vi "HFRR ADV v13.vi"() -> ()   [LabVIEW 2025] (continued)
              n2120 = String Subset(string=w2617, offset (0)=65, length (rest)=9 ("length (rest)")) -> (substring=w2638:string)
              n2121 = Fract/Exp String To Number(string=w2624) -> (number=w2621:dbl)  [unwired: 3 in, 1 out]
              n2122 = Fract/Exp String To Number(string=w2618) -> (number=w2616:dbl)  [unwired: 3 in, 1 out]
              n2123 = Fract/Exp String To Number(string=w2626) -> (number=w2625:dbl)  [unwired: 3 in, 1 out]
              n2124 = Fract/Exp String To Number(string=w2632) -> (number=w2629:dbl)  [unwired: 3 in, 1 out]
              n2125 = Fract/Exp String To Number(string=w2638) -> (number=w2635:dbl)  [unwired: 3 in, 1 out]
              n2126 = Add(x=w2635, y=0.0) -> (x+y=w2633:dbl)
            }
            n2127 = for {
              N: w2487 -> [_]
              tunnel: w2498 -> [w2578]
              tunnel: w2497 -> [w2577]
              tunnel: [w2567] -> w2456 mode=indexing
              tunnel: [w2565] -> w2454 mode=indexing
              tunnel: [w2566] -> w2450 mode=indexing
              tunnel: w2485 -> [_]
              tunnel: [w2559] -> w2452 mode=indexing
              tunnel: [w2555] -> w2434 mode=indexing
              tunnel: [w2551] -> w2410 mode=indexing
              tunnel: [w2548] -> w2391 mode=indexing
              tunnel: [w2544] -> w2350 mode=indexing
              (unwired) 9 ("length (rest)")
              (unwired) 9 ("length (rest)")
              (unwired) TRUE ("line mode (F)")
              n2128 = Read from Text File "Read File"(file (use dialog)=w2577, error in=w2578) -> (text=w2545:string)  [unwired: 2 in, 3 out]
              n2129 = local write "String 8"(w2545) -> ()
              n2130 = String Subset(string=w2545, offset (0)=85) -> (substring=w2547:string)  [unwired: 1 in]
              n2131 = String Subset(string=w2545, offset (0)=35, length (rest)=9 ("length (rest)")) -> (substring=w2568:string)
              n2132 = String Subset(string=w2545, offset (0)=55, length (rest)=9 ("length (rest)")) -> (substring=w2553:string)
              n2133 = String Subset(string=w2545, offset (0)=25) -> (substring=w2549:string)  [unwired: 1 in]
              n2134 = String Subset(string=w2545, offset (0)=15, length (rest)=9 ("length (rest)")) -> (substring=w2574:string)
              n2135 = String Subset(string=w2545, offset (0)=0, length (rest)=14 ("length (rest)")) -> (substring=w2571:string)
              n2136 = String Subset(string=w2545, offset (0)=45, length (rest)=9 ("length (rest)")) -> (substring=w2558:string)
              n2137 = String Subset(string=w2545, offset (0)=65, length (rest)=9 ("length (rest)")) -> (substring=w2564:string)
              n2138 = Fract/Exp String To Number(string=w2547) -> (number=w2544:dbl)  [unwired: 3 in, 1 out]
              n2139 = Fract/Exp String To Number(string=w2568) -> (number=w2566:dbl)  [unwired: 3 in, 1 out]
              n2140 = Fract/Exp String To Number(string=w2553) -> (number=w2551:dbl)  [unwired: 3 in, 1 out]
              n2141 = Fract/Exp String To Number(string=w2549) -> (number=w2548:dbl)  [unwired: 3 in, 1 out]
              n2142 = Fract/Exp String To Number(string=w2574) -> (number=w2565:dbl)  [unwired: 3 in, 1 out]
              n2143 = Fract/Exp String To Number(string=w2571) -> (number=w2567:dbl)  [unwired: 3 in, 1 out]
              n2144 = Fract/Exp String To Number(string=w2558) -> (number=w2555:dbl)  [unwired: 3 in, 1 out]
              n2145 = Fract/Exp String To Number(string=w2564) -> (number=w2561:dbl)  [unwired: 3 in, 1 out]
              n2146 = Add(x=w2561, y=0.0) -> (x+y=w2559:dbl)
            }
            n2147 = String To Path(string=w2404) -> (path=w2502:path)
            n2148 = String To Path(string=w2402) -> (path=w2496:path)
            n2149 = local read "Numeric 11"() -> (w2486:i32)
            n2150 = local read "Numeric 13"() -> (w2488:i32)
            n2151 = Open/Create/Replace File "Open File"(file path (use dialog)=w2502) -> (refnum out=w2500:refnum<file>, error out=w2499:errorcluster)  [unwired: 5 in, 1 out]
            n2152 = Open/Create/Replace File "Open File"(file path (use dialog)=w2496) -> (refnum out=w2495:refnum<file>, error out=w2494:errorcluster)  [unwired: 5 in, 1 out]
            n2153 = for {
              N: w2486 -> [_]
              tunnel: w2500 -> [w2615]
              tunnel: w2499 -> [w2614]
              tunnel: [w2604] -> w2466 mode=indexing
              tunnel: [w2602] -> w2464 mode=indexing
              tunnel: [w2603] -> w2459 mode=indexing
              tunnel: w2485 -> [_]
              tunnel: [w2596] -> w2461 mode=indexing
              tunnel: [w2592] -> w2437 mode=indexing
              tunnel: [w2588] -> w2412 mode=indexing
              tunnel: [w2584] -> w2393 mode=indexing
              tunnel: [w2579] -> w2351 mode=indexing
              (unwired) TRUE ("line mode (F)")
              n2154 = Read from Text File "Read File"(file (use dialog)=w2615, error in=w2614) -> (text=w2580:string)  [unwired: 2 in, 3 out]
              n2155 = local write "String 7"(w2580) -> ()
              n2156 = String Subset(string=w2580, offset (0)=85, length (rest)=9 ("length (rest)")) -> (substring=w2583:string)
              n2157 = String Subset(string=w2580, offset (0)=35, length (rest)=9 ("length (rest)")) -> (substring=w2605:string)
              n2158 = String Subset(string=w2580, offset (0)=55, length (rest)=9 ("length (rest)")) -> (substring=w2591:string)
              n2159 = String Subset(string=w2580, offset (0)=25, length (rest)=9 ("length (rest)")) -> (substring=w2585:string)
              n2160 = String Subset(string=w2580, offset (0)=45, length (rest)=9 ("length (rest)")) -> (substring=w2593:string)
              n2161 = String Subset(string=w2580, offset (0)=0, length (rest)=14 ("length (rest)")) -> (substring=w2608:string)
              n2162 = String Subset(string=w2580, offset (0)=15, length (rest)=9 ("length (rest)")) -> (substring=w2611:string)
              n2163 = String Subset(string=w2580, offset (0)=65, length (rest)=9 ("length (rest)")) -> (substring=w2597:string)
              n2164 = Fract/Exp String To Number(string=w2583) -> (number=w2579:dbl)  [unwired: 3 in, 1 out]
              n2165 = Fract/Exp String To Number(string=w2605) -> (number=w2603:dbl)  [unwired: 3 in, 1 out]
              n2166 = Fract/Exp String To Number(string=w2591) -> (number=w2588:dbl)  [unwired: 3 in, 1 out]
              n2167 = Fract/Exp String To Number(string=w2585) -> (number=w2584:dbl)  [unwired: 3 in, 1 out]
              n2168 = Fract/Exp String To Number(string=w2593) -> (number=w2592:dbl)  [unwired: 3 in, 1 out]
              n2169 = Fract/Exp String To Number(string=w2608) -> (number=w2604:dbl)  [unwired: 3 in, 1 out]
              n2170 = Fract/Exp String To Number(string=w2611) -> (number=w2602:dbl)  [unwired: 3 in, 1 out]
              n2171 = Fract/Exp String To Number(string=w2597) -> (number=w2600:dbl)  [unwired: 3 in, 1 out]
              n2172 = Add(x=w2600, y=0.0) -> (x+y=w2596:dbl)
            }
            n2173 = for {
              N: w2488 -> [_]
              tunnel: w2495 -> [w2543]
              tunnel: w2494 -> [w2542]
              tunnel: [w2532] -> w2448 mode=indexing
              tunnel: [w2531] -> w2441 mode=indexing
              tunnel: w2485 -> [_]
              tunnel: [w2520] -> w2446 mode=indexing
              tunnel: [w2525] -> w2443 mode=indexing
              tunnel: [w2521] -> w2433 mode=indexing
              tunnel: [w2516] -> w2408 mode=indexing
              tunnel: [w2512] -> w2389 mode=indexing
              tunnel: [w2507] -> w2349 mode=indexing
              (unwired) 1.0 ("x")
              (unwired) TRUE ("line mode (F)")
              n2174 = Read from Text File "Read File"(file (use dialog)=w2543, error in=w2542) -> (text=w2508:string)  [unwired: 2 in, 3 out]
              n2175 = local write "String 12"(w2508) -> ()
              n2176 = String Subset(string=w2508, offset (0)=85, length (rest)=9 ("length (rest)")) -> (substring=w2510:string)
              n2177 = String Subset(string=w2508, offset (0)=35, length (rest)=9 ("length (rest)")) -> (substring=w2533:string)
              n2178 = String Subset(string=w2508, offset (0)=55, length (rest)=9 ("length (rest)")) -> (substring=w2518:string)
              n2179 = String Subset(string=w2508, offset (0)=25, length (rest)=9 ("length (rest)")) -> (substring=w2514:string)
              n2180 = String Subset(string=w2508, offset (0)=45, length (rest)=9 ("length (rest)")) -> (substring=w2523:string)
              n2181 = String Subset(string=w2508, offset (0)=15, length (rest)=9 ("length (rest)")) -> (substring=w2539:string)
              n2182 = String Subset(string=w2508, offset (0)=0, length (rest)=14 ("length (rest)")) -> (substring=w2536:string)
              n2183 = String Subset(string=w2508, offset (0)=65, length (rest)=9 ("length (rest)")) -> (substring=w2526:string)
              n2184 = Fract/Exp String To Number(string=w2510) -> (number=w2507:dbl)  [unwired: 3 in, 1 out]
              n2185 = Fract/Exp String To Number(string=w2533) -> (number=w2531:dbl)  [unwired: 3 in, 1 out]
              n2186 = Fract/Exp String To Number(string=w2518) -> (number=w2516:dbl)  [unwired: 3 in, 1 out]
              n2187 = Fract/Exp String To Number(string=w2514) -> (number=w2512:dbl)  [unwired: 3 in, 1 out]
              n2188 = Fract/Exp String To Number(string=w2523) -> (number=w2521:dbl)  [unwired: 3 in, 1 out]
              n2189 = Fract/Exp String To Number(string=w2539) -> (number=w2520:dbl)  [unwired: 3 in, 1 out]
              n2190 = Fract/Exp String To Number(string=w2536) -> (number=w2532:dbl)  [unwired: 3 in, 1 out]
              n2191 = Fract/Exp String To Number(string=w2526) -> (number=w2529:dbl)  [unwired: 3 in, 1 out]
              n2192 = Add(x=w2529, y=0.0) -> (x+y=w2525:dbl)
            }
            n2193 = Delete From Array(array=w2391, index=0) -> (array with subset deleted=w2364:dbl[])  [unwired: 1 in, 1 out]
            n2194 = Delete From Array(array=w2454, index=0) -> (array with subset deleted=w2427:dbl[])  [unwired: 1 in, 1 out]
            n2195 = Delete From Array(array=w2434, index=0) -> (array with subset deleted=w2422:dbl[])  [unwired: 1 in, 1 out]
            n2196 = Delete From Array(array=w2452, index=0) -> (array with subset deleted=w2453:dbl[])  [unwired: 1 in, 1 out]
            n2197 = call-poly <vilib>:"Mean.vi"("X"=w2364) -> ("mean"=→"КОФ2 4":dbl)  [unwired: 1 out]
            n2198 = call-poly <vilib>:"Mean.vi"("X"=w2427) -> ("mean"=→"КОФ3":dbl)  [unwired: 1 out]
            n2199 = call-poly <vilib>:"Mean.vi"("X"=w2422) -> ("mean"=→"CP3":dbl)  [unwired: 1 out]
            n2200 = Delete From Array(array=w2416, index=0) -> (array with subset deleted=w2343:dbl[])  [unwired: 1 in, 1 out]
            n2201 = Delete From Array(array=w2355, index=0) -> (array with subset deleted=w2342:dbl[])  [unwired: 1 in, 1 out]
            n2202 = Delete From Array(array=w2395, index=0) -> (array with subset deleted=w2366:dbl[])  [unwired: 1 in, 1 out]
            n2203 = Delete From Array(array=w2473, index=0) -> (array with subset deleted=w2428:dbl[])  [unwired: 1 in, 1 out]
            n2204 = Delete From Array(array=w2439, index=0) -> (array with subset deleted=w2424:dbl[])  [unwired: 1 in, 1 out]
            "array w/ subset deleted" <- w2424
            n2205 = Delete From Array(array=w2470, index=0) -> (array with subset deleted=w2471:dbl[])  [unwired: 1 in, 1 out]
            n2206 = call-poly <vilib>:"Mean.vi"("X"=w2366) -> ("mean"=→"КОФ2 2":dbl)  [unwired: 1 out]
            n2207 = call-poly <vilib>:"Mean.vi"("X"=w2428) -> ("mean"=→"КОФ1":dbl)  [unwired: 1 out]
            n2208 = Bundle "Bundle"(w2343, w2342) -> (w2348:cluster{dbl[], dbl[]})  [unwired: 1 in]
            n2209 = Bundle "Bundle"(w2343, w2471) -> (w2335:cluster{dbl[], dbl[]})  [unwired: 1 in]
            n2210 = Delete From Array(array=w2350, index=0) -> (array with subset deleted=w2338:dbl[])  [unwired: 1 in, 1 out]
            n2211 = Delete From Array(array=w2351, index=0) -> (array with subset deleted=w2340:dbl[])  [unwired: 1 in, 1 out]
            n2212 = Delete From Array(array=w2461, index=0) -> (array with subset deleted=w2462:dbl[])  [unwired: 1 in, 1 out]
            n2213 = Delete From Array(array=w2349, index=0) -> (array with subset deleted=w2336:dbl[])  [unwired: 1 in, 1 out]
            n2214 = Delete From Array(array=w2443, index=0) -> (array with subset deleted=w2444:dbl[])  [unwired: 1 in, 1 out]
            n2215 = Delete From Array(array=w2468, index=0) -> (array with subset deleted=w2374:dbl[])  [unwired: 1 in, 1 out]
            n2216 = Delete From Array(array=w2414, index=0) -> (array with subset deleted=w2370:dbl[])  [unwired: 1 in, 1 out]
            n2217 = Delete From Array(array=w2450, index=0) -> (array with subset deleted=w2372:dbl[])  [unwired: 1 in, 1 out]
            n2218 = Delete From Array(array=w2410, index=0) -> (array with subset deleted=w2368:dbl[])  [unwired: 1 in, 1 out]
            n2219 = Delete From Array(array=w2459, index=0) -> (array with subset deleted=w2373:dbl[])  [unwired: 1 in, 1 out]
            n2220 = Delete From Array(array=w2412, index=0) -> (array with subset deleted=w2369:dbl[])  [unwired: 1 in, 1 out]
            n2221 = Delete From Array(array=w2393, index=0) -> (array with subset deleted=w2365:dbl[])  [unwired: 1 in, 1 out]
            n2222 = Delete From Array(array=w2437, index=0) -> (array with subset deleted=w2423:dbl[])  [unwired: 1 in, 1 out]
            n2223 = Delete From Array(array=w2464, index=0) -> (array with subset deleted=w2425:dbl[])  [unwired: 1 in, 1 out]
            n2224 = Delete From Array(array=w2441, index=0) -> (array with subset deleted=w2371:dbl[])  [unwired: 1 in, 1 out]
            n2225 = Delete From Array(array=w2408, index=0) -> (array with subset deleted=w2367:dbl[])  [unwired: 1 in, 1 out]
            n2226 = Delete From Array(array=w2389, index=0) -> (array with subset deleted=w2363:dbl[])  [unwired: 1 in, 1 out]
            n2227 = Delete From Array(array=w2433, index=0) -> (array with subset deleted=w2421:dbl[])  [unwired: 1 in, 1 out]
            n2228 = Delete From Array(array=w2446, index=0) -> (array with subset deleted=w2426:dbl[])  [unwired: 1 in, 1 out]
            n2229 = Delete From Array(array=w2456, index=0) -> (array with subset deleted=w2339:dbl[])  [unwired: 1 in, 1 out]
            n2230 = Delete From Array(array=w2466, index=0) -> (array with subset deleted=w2341:dbl[])  [unwired: 1 in, 1 out]
            n2231 = Delete From Array(array=w2448, index=0) -> (array with subset deleted=w2337:dbl[])  [unwired: 1 in, 1 out]
            n2232 = Bundle "Bundle"(w2343, w2374) -> (w2361:cluster{dbl[], dbl[]})  [unwired: 1 in]
            n2233 = Bundle "Bundle"(w2343, w2428) -> (w2362:cluster{dbl[], dbl[]})  [unwired: 1 in]
            n2234 = Bundle "Bundle"(w2374, w2370) -> (w2376:cluster{dbl[], dbl[]})  [unwired: 1 in]
            n2235 = Bundle "Bundle"(w2339, w2338) -> (w2346:cluster{dbl[], dbl[]})  [unwired: 1 in]
            n2236 = Bundle "Bundle"(w2372, w2368) -> (w2378:cluster{dbl[], dbl[]})  [unwired: 1 in]
            n2237 = Bundle "Bundle"(w2339, w2372) -> (w2482:cluster{dbl[], dbl[]})  [unwired: 1 in]
            n2238 = Bundle "Bundle"(w2339, w2368) -> (w2406:cluster{dbl[], dbl[]})  [unwired: 1 in]
            n2239 = Bundle "Bundle"(w2339, w2427) -> (w2492:cluster{dbl[], dbl[]})  [unwired: 1 in]
            n2240 = Bundle "Bundle"(w2339, w2422) -> (w2430:cluster{dbl[], dbl[]})  [unwired: 1 in]
            n2241 = Bundle "Bundle"(w2339, w2453) -> (w2477:cluster{dbl[], dbl[]})  [unwired: 1 in]
            n2242 = Bundle "Bundle"(w2373, w2369) -> (w2377:cluster{dbl[], dbl[]})  [unwired: 1 in]
            n2243 = Bundle "Bundle"(w2341, w2340) -> (w2347:cluster{dbl[], dbl[]})  [unwired: 1 in]
            n2244 = Bundle "Bundle"(w2341, w2373) -> (w2484:cluster{dbl[], dbl[]})  [unwired: 1 in]
            n2245 = Bundle "Bundle"(w2341, w2369) -> (w2407:cluster{dbl[], dbl[]})  [unwired: 1 in]
            n2246 = Bundle "Bundle"(w2341, w2423) -> (w2431:cluster{dbl[], dbl[]})  [unwired: 1 in]
            n2247 = Bundle "Bundle"(w2341, w2425) -> (w2493:cluster{dbl[], dbl[]})  [unwired: 1 in]
            n2248 = Bundle "Bundle"(w2341, w2462) -> (w2475:cluster{dbl[], dbl[]})  [unwired: 1 in]
            n2249 = Bundle "Bundle"(w2371, w2367) -> (w2379:cluster{dbl[], dbl[]})  [unwired: 1 in]
            n2250 = Bundle "Bundle"(w2337, w2336) -> (w2345:cluster{dbl[], dbl[]})  [unwired: 1 in]
            n2251 = Bundle "Bundle"(w2337, w2371) -> (w2483:cluster{dbl[], dbl[]})  [unwired: 1 in]
            n2252 = Bundle "Bundle"(w2337, w2367) -> (w2405:cluster{dbl[], dbl[]})  [unwired: 1 in]
            n2253 = Bundle "Bundle"(w2337, w2421) -> (w2429:cluster{dbl[], dbl[]})  [unwired: 1 in]
            n2254 = Bundle "Bundle"(w2337, w2426) -> (w2491:cluster{dbl[], dbl[]})  [unwired: 1 in]
            n2255 = Bundle "Bundle"(w2337, w2444) -> (w2476:cluster{dbl[], dbl[]})  [unwired: 1 in]
            n2256 = call-poly <vilib>:"Mean.vi"("X"=w2424) -> ("mean"=→"CP1":dbl)  [unwired: 1 out]
            n2257 = call-poly <vilib>:"Mean.vi"("X"=w2365) -> ("mean"=→"КОФ2 3":dbl)  [unwired: 1 out]
            n2258 = call-poly <vilib>:"Mean.vi"("X"=w2423) -> ("mean"=→"CP2":dbl)  [unwired: 1 out]
            n2259 = call-poly <vilib>:"Mean.vi"("X"=w2425) -> ("mean"=→"КОФ2":dbl)  [unwired: 1 out]
            n2260 = call-poly <vilib>:"Mean.vi"("X"=w2363) -> ("mean"=→"КОФ2 5":dbl)  [unwired: 1 out]
            n2261 = call-poly <vilib>:"Mean.vi"("X"=w2421) -> ("mean"=→"CP4":dbl)  [unwired: 1 out]
            n2262 = call-poly <vilib>:"Mean.vi"("X"=w2426) -> ("mean"=→"КОФ4":dbl)  [unwired: 1 out]
            n2263 = Bundle "Bundle"(w2343, w2370) -> (w2334:cluster{dbl[], dbl[]})  [unwired: 1 in]
            n2264 = Bundle "Bundle"(w2343, w2424) -> (w2357:cluster{dbl[], dbl[]})  [unwired: 1 in]
            n2265 = Build Array "Build Array"(w2334, w2357) -> (w2360:cluster{dbl[], dbl[]}[])
            "XY Graph 17" <- w2360
            n2266 = Build Array "Build Array"(w2348, w2347, w2346, w2345) -> (→"Frequency ( Hz )":cluster{dbl[], dbl[]}[])
            n2267 = Build Array "Build Array"(w2376, w2377, w2378, w2379) -> (→"Air Temp ( °C ) vs Humidity ( % RH )":cluster{dbl[], dbl[]}[])
            n2268 = Build Array "Build Array"(w2361, w2484, w2482, w2483) -> (→"Air Temperature  ( °C )":cluster{dbl[], dbl[]}[])
            n2269 = Build Array "Build Array"(w2334, w2407, w2406, w2405) -> (→"Humidity ( %RH )":cluster{dbl[], dbl[]}[])
            n2270 = Build Array "Build Array"(w2362, w2493, w2492, w2491) -> (→"Coefficient Of Friction":cluster{dbl[], dbl[]}[])
            n2271 = Build Array "Build Array"(w2357, w2431, w2430, w2429) -> (→"Sample Temperature ( °C )":cluster{dbl[], dbl[]}[])
            n2272 = Build Array "Build Array"(w2335, w2475, w2477, w2476) -> (→"XY Graph 13":cluster{dbl[], dbl[]}[])
            n2273 = Bundle "Bundle"(w2343, w2366) -> (w2388:cluster{dbl[], dbl[]})  [unwired: 1 in]
            n2274 = Bundle "Bundle"(w2339, w2364) -> (w2386:cluster{dbl[], dbl[]})  [unwired: 1 in]
            n2275 = Bundle "Bundle"(w2341, w2365) -> (w2387:cluster{dbl[], dbl[]})  [unwired: 1 in]
            n2276 = Bundle "Bundle"(w2337, w2363) -> (w2385:cluster{dbl[], dbl[]})  [unwired: 1 in]
            n2277 = Build Array "Build Array"(w2388, w2387, w2386, w2385) -> (→"Stroke ( mm )":cluster{dbl[], dbl[]}[])
            n2278 = local write "XY Graph 16"(w2360) -> ()
          }
          frame #2 {
          }
          frame #3 {
            n2279 = local write "Numeric 8"(0 ("Numeric 8")) -> ()
            n2280 = local write "Numeric 11"(0 ("Numeric 11")) -> ()
            n2281 = local write "Numeric 12"(0 ("Numeric 12")) -> ()
            n2282 = local write "Numeric 13"(0 ("Numeric 13")) -> ()
            n2283 = property on="OPEN" class="Bool (strict)"("Visible"=TRUE) -> ()  [unwired: 2 in, 2 out]
            n2284 = local read "String Control 2"() -> (w2660:string)
            n2285 = local read "String Control 4"() -> (w2659:string)
            n2286 = local read "String Control 6"() -> (w2658:string)
            n2287 = local read "String Control 8"() -> (w2657:string)
            n2288 = Match Pattern(string=w2660, regular expression="Samples / cycle :- ") -> (after substring=w2674:string)  [unwired: 1 in, 3 out]
            n2289 = Match Pattern(string=w2660, regular expression="Frequency :- ") -> (after substring=w2693:string)  [unwired: 1 in, 3 out]
            n2290 = Match Pattern(string=w2659, regular expression="Samples / cycle :- ") -> (after substring=w2670:string)  [unwired: 1 in, 3 out]
            n2291 = Match Pattern(string=w2659, regular expression="Frequency :- ") -> (after substring=w2688:string)  [unwired: 1 in, 3 out]
            n2292 = Match Pattern(string=w2658, regular expression="Samples / cycle :- ") -> (after substring=w2666:string)  [unwired: 1 in, 3 out]
            n2293 = Match Pattern(string=w2658, regular expression="Frequency :- ") -> (after substring=w2683:string)  [unwired: 1 in, 3 out]
            n2294 = Match Pattern(string=w2657, regular expression="Samples / cycle :- ") -> (after substring=w2662:string)  [unwired: 1 in, 3 out]
            n2295 = Match Pattern(string=w2657, regular expression="Frequency :- ") -> (after substring=w2678:string)  [unwired: 1 in, 3 out]
            n2296 = String Subset(string=w2674, length (rest)=6 ("length (rest)")) -> (substring=w2676:string)  [unwired: 1 in]
            n2297 = String Subset(string=w2693, length (rest)=9 ("length (rest)")) -> (substring=w2695:string)  [unwired: 1 in]
            n2298 = String Subset(string=w2670, length (rest)=6 ("length (rest)")) -> (substring=w2672:string)  [unwired: 1 in]
            n2299 = String Subset(string=w2688, length (rest)=9 ("length (rest)")) -> (substring=w2690:string)  [unwired: 1 in]
            n2300 = String Subset(string=w2666, length (rest)=6 ("length (rest)")) -> (substring=w2668:string)  [unwired: 1 in]
            n2301 = String Subset(string=w2683, length (rest)=9 ("length (rest)")) -> (substring=w2685:string)  [unwired: 1 in]
            n2302 = String Subset(string=w2662, length (rest)=6 ("length (rest)")) -> (substring=w2664:string)  [unwired: 1 in]
            n2303 = String Subset(string=w2678, length (rest)=9 ("length (rest)")) -> (substring=w2680:string)  [unwired: 1 in]
            n2304 = Fract/Exp String To Number(string=w2676) -> (number=w2656:dbl)  [unwired: 3 in, 1 out]
            n2305 = Fract/Exp String To Number(string=w2695) -> (number=w2696:dbl)  [unwired: 3 in, 1 out]
            n2306 = Fract/Exp String To Number(string=w2672) -> (number=w2655:dbl)  [unwired: 3 in, 1 out]
            n2307 = Fract/Exp String To Number(string=w2690) -> (number=w2691:dbl)  [unwired: 3 in, 1 out]
            n2308 = Fract/Exp String To Number(string=w2668) -> (number=w2654:dbl)  [unwired: 3 in, 1 out]
            n2309 = Fract/Exp String To Number(string=w2685) -> (number=w2686:dbl)  [unwired: 3 in, 1 out]
            n2310 = Fract/Exp String To Number(string=w2664) -> (number=w2653:dbl)  [unwired: 3 in, 1 out]
            n2311 = Fract/Exp String To Number(string=w2680) -> (number=w2681:dbl)  [unwired: 3 in, 1 out]
            n2312 = local write "sample1"(w2656) -> ()
            n2313 = local write "freq1"(w2696) -> ()
            n2314 = local write "sample2"(w2655) -> ()
            n2315 = local write "freq2"(w2691) -> ()
            n2316 = local write "sample3"(w2654) -> ()
            n2317 = local write "freq3"(w2686) -> ()
            n2318 = local write "sample4"(w2653) -> ()
            n2319 = local write "freq 4"(w2681) -> ()
          }
        }
      }
    }
    n2320 = case shown="True" w2143 {
      selector: w2143 -> [_ w2272]
      frame False {
      }
      frame True {
        n2321 = Not(x=w2272) -> (.not. x?=w2268:bool)
        n2322 = local write "service 3"(w2268) -> ()
        n2323 = local write "OPEN 6"(w2268) -> ()
        n2324 = call <vilib>:"System Exec.vi"("wait until completion? (T)"=TRUE, "command line"="C:\\LAB-IQ\\Scar View.exe") -> ("error out"=→"error out 5":errorcluster)  [unwired: 6 in, 3 out]
      }
    }
    n2325 = case shown="\"Acquire\", Default" w2155 {
      frame "Acquire", Default {
        w3195 = 0.2 ("y")
        w3200 = 1.0 ("y")
        w3201 = 0.8 ("y")
        # "Elapsed time\ncof\nstroke\nAir temp\nTemp\nHumidity"
        n2326 = disable-structure shown="Disabled" {
          frame Disabled {
            n2327 = local read "Flag"() -> (w3218:dbl)
            n2328 = local read "RUN"() -> (w3215:bool)
            n2329 = Not(x=w3215) -> (.not. x?=w3214:bool)
            n2330 = Equal?(x=w3218, y=10.0) -> (x = y?=w3216:bool)
            n2331 = And(x=w3216, y=w3214) -> (x .and. y?=w3213:bool)
            n2332 = case shown="True" w3213 {
              frame False {
              }
              frame True {
                w3219 = FALSE ("Heater Button")
                n2333 = local write "Humidity"(w3219) -> ()
                n2334 = local write "Heater Button"(w3219) -> ()
              }
            }
          }
          frame Enabled {
          }
        }
        n2335 = disable-structure shown="Disabled" {
          frame Disabled {
            n2336 = case shown="True" {
              selector: _ -> [_ _]
              frame False {
              }
              frame True {
                w3310 = TRUE ("Heater")
                n2337 = local write "Humidity"(w3310) -> ()
                n2338 = local write "Heater Button"(w3310) -> ()
                n2339 = local read "TEST STANDARD"() -> (w3313:T3)
                n2340 = local read "TEST STANDARD"() -> (w3308:T3)
                n2341 = Equal?(x=w3313, y=enum16{"ASTM D6079", "ISO 12156", "Custom"}."ISO 12156" ("Test Standard")) -> (x = y?=w3311:bool)
                n2342 = Equal?(x=w3308, y=enum16{"ASTM D6079", "ISO 12156", "Custom"}."ASTM D6079" ("Test Standard")) -> (x = y?=w3307:bool)
                n2343 = case shown="True" w3311 {
                  frame False {
                  }
                  frame True {
                    n2344 = local write "Heater"(TRUE ("Heater")) -> ()
                    n2345 = local write "airtempflg"(FALSE ("airtempflg")) -> ()
                  }
                }
                n2346 = case shown="True" w3307 {
                  frame False {
                  }
                  frame True {
                    n2347 = local write "Heater"(FALSE ("Heater")) -> ()
                    n2348 = local write "airtempflg"(TRUE ("airtempflg")) -> ()
                  }
                }
              }
            }
          }
          frame Enabled {
          }
        }
        n2349 = stacked-sequence {
          frame #0 {
            n2350 = case shown="True" "RST FF" {
              frame False {
              }
              frame True {
                w3376 = 0.0 ("X Scale.Range:Maximum")
                n2351 = property on="Frictional Force ( N )" class="WFChart (strict)"("XScale.Maximum"=600.0 ("X Scale.Range:Maximum"), "XScale.Minimum"=w3376, "YScale.Maximum"=10.0 ("Y Scale.Range:Maximum"), "YScale.Minimum"=w3376) -> ()  [unwired: 2 in, 2 out]
              }
            }
          }
          frame #1 {
            n2352 = case shown="True" "RST TEMP" {
              frame False {
              }
              frame True {
                n2353 = property on="Temperature ( Deg C )" class="WFChart (strict)"("XScale.Minimum"=0.0 ("X Scale.Range:Minimum"), "XScale.Maximum"=600.0 ("X Scale.Range:Maximum"), "YScale.Minimum"=0.0 ("Y Scale.Range:Minimum"), "YScale.Maximum"=100.0 ("Y Scale.Range:Maximum")) -> ()  [unwired: 2 in, 2 out]
              }
            }
          }
          frame #2 {
            n2354 = case shown="True" "RSTCOF" {
              frame False {
              }
              frame True {
                n2355 = property on="Coefficient of Friction" class="WFChart (strict)"("XScale.Minimum"=0.0 ("X Scale.Range:Minimum"), "XScale.Maximum"=600.0 ("X Scale.Range:Maximum"), "YScale.Maximum"=1.0 ("X Scale.Range:Minimum"), "YScale.Minimum"=0.0 ("X Scale.Range:Minimum")) -> ()  [unwired: 2 in, 2 out]
              }
            }
          }
          frame #3 {
            n2356 = case shown="True" "RSTCOF 2" {
              frame False {
              }
              frame True {
                (unwired) 100.0 ("Y Scale.Range:Maximum")
                (unwired) 0.0 ("Y Scale.Range:Minimum")
                (unwired) 600.0 ("X Scale.Range:Maximum")
                (unwired) 0.0 ("X Scale.Range:Minimum")
              }
            }
          }
          frame #4 {
            n2357 = case shown="True" "RSTCOF 3" {
              frame False {
              }
              frame True {
                n2358 = property on="Electrical Contact Resistance ( % )" class="WFChart (strict)"("XScale.Minimum"=0.0 ("X Scale.Range:Minimum"), "XScale.Maximum"=600.0 ("X Scale.Range:Maximum"), "YScale.Minimum"=0.0 ("Y Scale.Range:Minimum"), "YScale.Maximum"=100.0 ("Y Scale.Range:Maximum")) -> ()  [unwired: 2 in, 2 out]
              }
            }
          }
        }
        n2359 = disable-structure shown="Disabled" {
          frame Disabled {
            n2360 = case shown="True" {
              selector: _ -> [_ _]
              frame False {
              }
              frame True {
                n2361 = local read "zflag 2"() -> (w3277:dbl)
                n2362 = local read "yflag"() -> (w3279:dbl)
                n2363 = Equal?(x=w3279, y=2.0 ("tflag")) -> (x = y?=w3281:bool)
                n2364 = Equal?(x=w3277, y=3.0 ("tflag")) -> (x = y?=w3280:bool)
                n2365 = And(x=w3281, y=w3280) -> (x .and. y?=w3275:bool)
                n2366 = case shown="True" w3275 {
                  frame False {
                  }
                  frame True {
                    w3306 = 0.0 ("zflag")
                    n2367 = local write "zflag"(w3306) -> ()
                    n2368 = local write "zflag 2"(w3306) -> ()
                    n2369 = Delete(path (use dialog)=path "C:/LAB-IQ-NXT/WO 2449 TT.sig" ("file path (dialog if empty)")) -> (deleted path=w3305:path)  [unwired: 4 in, 2 out]
                    n2370 = Delete(path (use dialog)=path "C:/LAB-IQ-NXT/WO 2449 TRH.sig" ("file path (dialog if empty)")) -> (deleted path=w3300:path)  [unwired: 4 in, 2 out]
                    n2371 = local read "SEN.RUN HRS"() -> (w3292:dbl)
                    n2372 = local read "SENSOR TIME"() -> (w3290:dbl)
                    n2373 = call <vilib>:"compatOverwrite.vi"("overwrite (F)"=TRUE) -> ("overwrite?"=w3282:T26)
                    n2374 = call <vilib>:"compatOverwrite.vi"("overwrite (F)"=TRUE) -> ("overwrite?"=w3286:T26)
                    n2375 = local read "Total No. of Tests"() -> (w3293:dbl)
                    n2376 = Add(x=w3290, y=w3292) -> (x+y=w3291:dbl)
                    "SEN.RUN HRS" <- w3291
                    n2377 = Open/Create/Replace File(file path (use dialog)=w3305, operation (0:open)=w3282) -> (refnum out=w3283:refnum<file>, error out=w3284:errorcluster)  [unwired: 4 in, 1 out]
                    n2378 = Open/Create/Replace File(file path (use dialog)=w3300, operation (0:open)=w3286) -> (refnum out=w3287:refnum<file>, error out=w3288:errorcluster)  [unwired: 4 in, 1 out]
                    n2379 = Deny Access(4:w3284, 6:T24."deny none" ("deny mode (2)"), 7:w3283) -> (3:w3304:refnum<file>)  [unwired: 1 out]
                    n2380 = Deny Access(4:w3288, 6:T24."deny none" ("deny mode (2)"), 7:w3287) -> (3:w3296:refnum<file>)  [unwired: 1 out]
                    n2381 = Number To Decimal String(number=w3293) -> (decimal integer string=w3301:string)  [unwired: 1 in]
                    n2382 = Number To Decimal String(number=w3291) -> (decimal integer string=w3297:string)  [unwired: 1 in]
                    n2383 = Write to Binary File(file (use dialog)=w3304, data=w3301, 5:FALSE ("prepend array or string size? (T)")) -> ()  [unwired: 3 in, 3 out]
                    n2384 = Write to Binary File(file (use dialog)=w3296, data=w3297, 5:FALSE ("prepend array or string size? (T)")) -> ()  [unwired: 3 in, 3 out]
                  }
                }
              }
            }
          }
          frame Enabled {
          }
        }
        n2385 = local read "RUN"() -> (w3204:bool)
        n2386 = local read "run replace"() -> (w3208:bool)
        n2387 = local read "run replace"() -> (w3207:bool)
        n2388 = case shown="True" w3204 {
          frame False {
            n2389 = local write "run replace"(FALSE ("run replace")) -> ()
          }
          frame True {
            "run replace" <- TRUE ("run replace")
          }
        }
        n2390 = local read "RUN"() -> (w3212:bool)
        n2391 = local read "Set Temp"() -> (w3174:dbl)
        n2392 = local read "SetTemp"() -> (w3176:dbl)
        n2393 = case shown="False" w3212 {
          tunnel: [FALSE ("TEST RUNNING") TRUE ("TEST RUNNING")] -> w3211
          frame False {
            w3395 = 0.0 ("Flag")
            n2394 = local write "Elapsed time"(0.0 ("elapsedtime")) -> ()
            n2395 = local write "Time Remaining"(w3395) -> ()
            n2396 = local write "Flag"(w3395) -> ()
            n2397 = local write "Remaining Time"(w3395) -> ()
          }
          frame True {
            n2398 = local write "Flag"(10.0 ("Flag")) -> ()
          }
        }
        n2399 = case shown="False" w3208 {
          frame False {
            n2400 = local read "zflag"() -> (→"zflag 2":dbl)
            n2401 = local write "yflag"(2.0 ("tflag")) -> ()
            n2402 = local write "FLAG 4"(0.0 ("FLAG")) -> ()
          }
          frame True {
            n2403 = local write "yflag"(1.0 ("tflag")) -> ()
            n2404 = local write "zflag"(3.0 ("zflag")) -> ()
          }
        }
        n2405 = local read "acq 2"() -> (w3206:bool)
        n2406 = local read "AIR TEMP"() -> (w3169:dbl)
        n2407 = local read "Amb temp"() -> (w3173:dbl)
        n2408 = case shown="True" "Save & Continue" {
          frame False {
          }
          frame True {
            "acq 2" <- TRUE ("acq 2")
          }
        }
        n2409 = local read "Set Rh"() -> (w3175:dbl)
        n2410 = Add(x=w3176, y=w3201) -> (x+y=w3202:dbl)
        n2411 = Subtract(x=w3176, y=w3201) -> (x-y=w3203:dbl)
        n2412 = Add(x=w3174, y=w3195) -> (x+y=w3196:dbl)
        n2413 = Subtract(x=w3174, y=w3195) -> (x-y=w3197:dbl)
        n2414 = And(x=w3206, y=w3207) -> (x .and. y?=w3205:bool)
        n2415 = Greater Or Equal?(x=w3169, y=15.0) -> (x >= y?=w3170:bool)
        "powstat" <- w3170
        n2416 = local read "Humidity ( %RH )"() -> (w3172:dbl)
        n2417 = case shown="True" "Save & Continue" {
          frame False {
          }
          frame True {
            n2418 = while {
              tunnel: "0123456789abcdefghijklmnopqrstuvwxyzABCDEFGHIJKLMNOPQRSTUVWXYZ" ("string 2") -> [w3366]
              shift-right: [w3364] -> w3359
              shift-left: "" -> [w3363]
              i -> [w3373]
              stop <- w3372 stop-if-true
              n2419 = Random Number (0-1)() -> (number: 0 to 1=w3367:dbl)
              n2420 = Multiply(x=w3367, y=62.0) -> (x*y=w3369:dbl)
              n2421 = Decrement(x="Length") -> (x-1=w3362:i16)
              n2422 = To Word Integer(number=w3369) -> (16bit integer=w3370:i16)
              n2423 = String Subset(string=w3366, offset (0)=w3370, length (rest)=1 ("length (rest)")) -> (substring=w3365:string)
              n2424 = Greater Or Equal?(x=w3373, y=w3362) -> (x >= y?=w3372:bool)
              n2425 = Concatenate Strings(w3365, w3363) -> (w3364:string)
            }
            n2426 = local write "UUID"(w3359) -> ()
          }
        }
        n2427 = In Range and Coerce(upper limit=w3202, x=w3173, lower limit=w3203) -> (In Range?=w3192:bool)  [unwired: 1 out]
        n2428 = Add(x=w3175, y=w3200) -> (x+y=w3199:dbl)
        n2429 = Subtract(x=w3175, y=w3200) -> (x-y=w3198:dbl)
        n2430 = local read "TEMP"() -> (w3171:dbl)
        n2431 = case shown="True" "Save & Continue" {
          frame False {
          }
          frame True {
            n2432 = local read "Operator ID"() -> (w3715:string)
            n2433 = local read "FILE"() -> (w3721:string)
            n2434 = String Length(string=w3721) -> (length=w3719:i32)
            n2435 = String Length(string=w3715) -> (length=w3716:i32)
            n2436 = Greater?(x=w3719, y=0) -> (0:w3718:bool)
            n2437 = Greater?(x=w3716, y=0) -> (0:w3714:bool)
            n2438 = And(x=w3718, y=w3714) -> (x .and. y?=w3713:bool)
            n2439 = case shown="True" w3713 {
              frame False {
                n2440 = stacked-sequence {
                  frame #0 {
                    n2441 = One Button Dialog(message="Please Enter a File Name and Operator ID to save data !", button name ("OK")="Ok") -> ()  [unwired: 1 out]
                  }
                  frame #1 {
                    n2442 = local write "Save & Continue"(FALSE ("OK Button")) -> ()
                  }
                }
                n2443 = local write "Save & Continue"(FALSE ("OK Button")) -> ()
              }
              frame True {
                n2444 = stacked-sequence {
                  frame #0 {
                    n2445 = local read "FILE"() -> (w3727:string)
                    n2446 = call "file check.vi"("file name in"=w3727) -> ("file name out"=w3726:string)  [unwired: 9 in, 1 out]
                    n2447 = call <vilib>:"Application Directory.vi"() -> ("Application Directory"=w3737:path)
                    n2448 = Build Path(base path=w3737, name or relative path="data") -> (appended path=w3736:path)
                    n2449 = call <vilib>:"Trim Whitespace.vi"("string"=w3726) -> ("trimmed string"=w3734:string)  [unwired: 1 in]
                    n2450 = call <vilib>:"Trim Whitespace.vi"("string"=w3726) -> ("trimmed string"=w3735:string)  [unwired: 1 in]
                    n2451 = List Folder(path=w3736) -> (folder names=w3732:string[])  [unwired: 3 in, 3 out]
                    n2452 = Match Pattern(string=w3734, regular expression="_(") -> (before substring=w3731:string)  [unwired: 1 in, 3 out]
                    n2453 = for {
                      tunnel: w3732 -> [w3746] mode=indexing
                      tunnel: w3731 -> [w3744]
                      shift-right: [w3742] -> w3729
                      shift-left: bool[] [] -> [w3743]
                      n2454 = Match Pattern(string=w3746, regular expression="_(") -> (before substring=w3745:string)  [unwired: 1 in, 3 out]
                      n2455 = Equal?(x=w3745, y=w3744) -> (x = y?=w3741:bool)
                      n2456 = case shown="True" w3741 {
                        tunnel: w3741 -> [_ w3749]
                        tunnel: w3743 -> [w3748 w3751]
                        tunnel: [w3748 w3750] -> w3742
                        frame False {
                        }
                        frame True {
                          n2457 = Insert Into Array(array=w3751, new element=w3749) -> (w3750:bool[])  [unwired: 1 in]
                        }
                      }
                    }
                    n2458 = Equal?(x=w3732, y=w3731) -> (x = y?=w3740:bool[])
                    n2459 = Or Array Elements(Boolean array=w3740) -> (logical OR=w3739:bool)
                    n2460 = Array Size(array=w3729) -> (size(s)=w3728:i32)
                    n2461 = case shown="True" w3739 {
                      tunnel: w3735 -> [_ w3759]
                      tunnel: w3728 -> [_ w3752]
                      frame False {
                      }
                      frame True {
                        n2462 = Number To Decimal String(number=w3752) -> (decimal integer string=w3755:string)  [unwired: 1 in]
                        n2463 = Search/Split String(string=w3759, search string/char (-)="_(" ("regular expression")) -> (substring before match=w3757:string)  [unwired: 1 in, 2 out]
                        n2464 = Concatenate Strings(w3757, "_(" ("regular expression"), w3755, ")" ("regular expression")) -> (w3753:string)
                        n2465 = local write "FILE"(w3753) -> ()
                      }
                    }
                  }
                  frame #1 {
                    w3761 = 0.0
                    w3774 = cluster{"y":dbl, dbl, "y":dbl}[] [] ("History Data")
                    w3775 = FALSE ("Heater Button")
                    (unwired) ")!" ("string")
                    (unwired) ")" ("string")
                    w3773 = dbl[] [] ("History Data")
                    w3779 = "\r"
                    # "C:\\WinDucom\\Data\\"
                    # "C:\\LAB-IQ-NXT\\data"
                    n2466 = local write "Humidity ( %RH )"(w3761) -> ()
                    n2467 = local write "Frequency ( Hz )"(w3761) -> ()
                    n2468 = local write "Stroke 3"(w3761) -> ()
                    n2469 = local write "speedop"(0.0 ("PIDclk 2")) -> ()
                    n2470 = local write "Set Temp 2"(65.0 ("Set Temp 2")) -> ()
                    n2471 = local write "AIR TEMP"(w3761) -> ()
                    n2472 = local write "clk"(0.0 ("clk")) -> ()
                    n2473 = local write "Stroke 4"(w3761) -> ()
                    n2474 = local write "Stroke"(w3761) -> ()
                    n2475 = local write "COF 3"(w3761) -> ()
                    n2476 = local write "COF 2"(w3761) -> ()
                    n2477 = local write "TEMP"(w3761) -> ()
                    n2478 = local write "ecr 3"(w3761) -> ()
                    n2479 = local write "FF 3"(w3761) -> ()
                    n2480 = local write "FF 2"(w3761) -> ()
                    n2481 = property on="Humidity ( %RH )" class="WFChart (strict)"("History Data"=w3773) -> ()  [unwired: 2 in, 2 out]
                    n2482 = property on="Coefficient of Friction" class="WFChart (strict)"("History Data"=w3773) -> ()  [unwired: 2 in, 2 out]
                    n2483 = property on="Coefficient of Friction" class="WFChart (strict)"("History Data"=w3773) -> ()  [unwired: 2 in, 2 out]
                    n2484 = property on="Frictional Force ( N )" class="WFChart (strict)"("History Data"=w3773) -> ()  [unwired: 2 in, 2 out]
                    n2485 = property on="Electrical Contact Resistance ( % )" class="WFChart (strict)"("History Data"=w3773) -> ()  [unwired: 2 in, 2 out]
                    n2486 = property on="Electrical Contact Resistance ( % )" class="WFChart (strict)"("History Data"=w3773) -> ()  [unwired: 2 in, 2 out]
                    n2487 = property on="Temperature ( Deg C )" class="WFChart (strict)"("History Data"=w3773) -> ()  [unwired: 2 in, 2 out]
                    n2488 = property on="Frictional Force ( N )" class="WFChart (strict)"("History Data"=w3773) -> ()  [unwired: 2 in, 2 out]
                    n2489 = property on="Coefficient of Friction" class="WFChart (strict)"("History Data"=w3773) -> ()  [unwired: 2 in, 2 out]
                    n2490 = property on="Frictional Force ( N )" class="WFChart (strict)"("History Data"=w3773) -> ()  [unwired: 2 in, 2 out]
                    n2491 = property on="Electrical Contact Resistance ( % )" class="WFChart (strict)"("History Data"=w3773) -> ()  [unwired: 2 in, 2 out]
                    n2492 = property on="Temperature ( Deg C )" class="WFChart (strict)"("History Data"=w3773) -> ()  [unwired: 2 in, 2 out]
                    n2493 = property on="Humidity ( %RH )" class="WFChart (strict)"("History Data"=w3773) -> ()  [unwired: 2 in, 2 out]
                    n2494 = property on="Stroke ( mm )" class="WFChart (strict)"("History Data"=w3774) -> ()  [unwired: 2 in, 2 out]
                    n2495 = property on="Stroke ( mm )" class="WFChart (strict)"("History Data"=w3774) -> ()  [unwired: 2 in, 2 out]
                    n2496 = local write "Humidity"(w3775) -> ()
                    n2497 = local write "Heater Button"(w3775) -> ()
                    n2498 = local read "FILE"() -> (w3769:string)
                    n2499 = disable-structure shown="Enabled" {
                      disable-tunnel: [w3814 _] -> w3760
                      frame Enabled {
                        n2500 = local read "NORMAL LOAD"() -> (w3814:dbl)
                      }
                      frame Disabled {
                      }
                    }
                    n2501 = call "file check.vi"("file name in"=w3769) -> ("error out"=w3772:errorcluster, "file name out"=w3766:string)  [unwired: 9 in]
                    n2502 = call "FILE PATH CREATION.vi"("error in"=w3772, "FILE NAME :"=w3766) -> ("FILE OUT"=w3765:path)  [unwired: 8 in, 1 out]
                    n2503 = Concatenate Strings(w3766, ".dgf" ("Substring")) -> (w3771:string)
                    n2504 = Concatenate Strings(w3766, ".duf" ("Substring")) -> (w3767:string)
                    n2505 = Multiply(x=w3760, y=1.0) -> (x*y=w3793:dbl)
                    n2506 = Build Path(base path=w3765, name or relative path=w3771) -> (appended path=w3764:path)
                    n2507 = Build Path(base path=w3765, name or relative path=w3767) -> (appended path=w3763:path)
                    n2508 = Number To Fractional String(number=w3793, width (-)=i16 5, precision (6)=i16 2) -> (F-format string=w3801:string)  [unwired: 1 in]
                    n2509 = local read "Fuel Discription :"() -> (w3789:string)
                    n2510 = local read "Batch Ref Num :"() -> (w3777:string)
                    n2511 = Get Date/Time String(date format (0)=enum16{"short", "long", "abbreviated"}."short") -> (date string=w3812:string, time string=w3809:string)  [unwired: 2 in]
                    n2512 = local read "Remarks :"() -> (w3788:string)
                    n2513 = Concatenate Strings("Load :- " ("Substring"), w3801, " grams ," ("Substring")) -> (w3800:string)
                    n2514 = local read "String 41"() -> (w3780:string)
                    n2515 = Concatenate Strings(w3789) -> (w3790:string)
                    n2516 = Concatenate Strings(w3777) -> (w3776:string)
                    n2517 = Concatenate Strings("tested by") -> (w3784:string)
                    n2518 = Concatenate Strings("(" ("Substring"), w3812, ")" ("Substring"), w3809) -> (w3782:string)
                    "concatenated string" <- w3782
                    n2519 = Concatenate Strings(w3788, "," ("string")) -> (w3787:string)
                    n2520 = Concatenate Strings("  TIME;      COF;       STROKE;     AIR TEMP;  TEMP;  HUMIDITY;  ECR; PID-OUT; FREQUENCY" ("Substring"), "\r") -> (w3796:string)
                    n2521 = Concatenate Strings(w3780, w3779, "Fuel Discription :-" ("Substring"), w3790, w3779, w3800, w3779, "Batch Ref Num :-" ("Substring"), w3776, w3779, " Remarks :- " ("Substring"), w3787, w3779, " Date :- " ("Substring"), w3782, w3779, "Tested By :-" ("Substring"), w3784) -> (w3794:string)
                    "REMARKS" <- w3794
                    n2522 = call <vilib>:"Write Characters To File.vi"("append to file? (new file:F)"=FALSE, "character string"=w3796, "file path (dialog if empty)"=w3764) -> ()  [unwired: 2 in, 1 out]
                    n2523 = call <vilib>:"Write Characters To File.vi"("append to file? (new file:F)"=FALSE, "character string"=w3794, "file path (dialog if empty)"=w3763) -> ()  [unwired: 2 in, 1 out]
                  }
                  frame #2 {
                    n2524 = local write "Cycles elapsed"(0 ("Cycles elapsed")) -> ()
                    n2525 = local write "cyclecount"(0 ("cyclecount")) -> ()
                    n2526 = local write "Save & Continue"(FALSE ("OK")) -> ()
                    n2527 = local write "autostrtflg"(TRUE ("autostrtflg")) -> ()
                    n2528 = local write "Save"(FALSE ("Save")) -> ()
                    n2529 = Get Date/Time In Seconds() -> (seconds since 1Jan1904=w3819:timestamp)
                    n2530 = To Double Precision Float(number=w3819) -> (double precision float=w3818:dbl)
                    n2531 = local write "acq timer"(w3818) -> ()
                    n2532 = One Button Dialog(message="Please ensure sample is mounted properly and machine is ready in all aspects for testing !", button name ("OK")="Ok") -> ()  [unwired: 1 out]
                  }
                  frame #3 {
                    n2533 = stacked-sequence {
                      frame #0 {
                        n2534 = local write "Main Dashboard Buttons"(T1."Dashboard" ("Main Dashboard Buttons")) -> ()
                        n2535 = local write "Main Tab"(T2."Acquire" ("Main Tab")) -> ()
                      }
                      frame #1 {
                        n2536 = local write "EVENT LOG"("" ("EVENT LOG")) -> ()
                      }
                      frame #2 {
                        n2537 = Wait (ms)(milliseconds to wait=u32 50) -> ()  [unwired: 1 out]
                      }
                      frame #3 {
                        n2538 = disable-structure shown="Disabled" {
                          frame Disabled {
                            n2539 = local read "EVENT LOG"() -> (w3831:string)
                            n2540 = call "Event Log.vi"("Content"="Test Details", "EVENT LOG"=w3831) -> ("EVENT LOG"=w3830:string)  [unwired: 8 in, 1 out]
                            n2541 = local write "EVENT LOG"(w3830) -> ()
                          }
                          frame Enabled {
                          }
                        }
                      }
                      frame #4 {
                        n2542 = Wait (ms)(milliseconds to wait=u32 50) -> ()  [unwired: 1 out]
                      }
                      frame #5 {
                        n2543 = local read "FILE"() -> (w3833:string)
                        n2544 = Concatenate Strings("File Name :" ("Content"), w3833) -> (w3834:string)
                        n2545 = local read "EVENT LOG"() -> (w3837:string)
                        n2546 = call "Event Log.vi"("Content"=w3834, "EVENT LOG"=w3837) -> ("EVENT LOG"=w3836:string)  [unwired: 8 in, 1 out]
                        n2547 = local write "EVENT LOG"(w3836) -> ()
                      }
                      frame #6 {
                        n2548 = Wait (ms)(milliseconds to wait=u32 50) -> ()  [unwired: 1 out]
                      }
                      frame #7 {
                        n2549 = local read "Batch Ref Num :"() -> (w3839:string)
                        n2550 = Concatenate Strings("Batch Ref No :" ("Content"), w3839) -> (w3840:string)
                        n2551 = local read "EVENT LOG"() -> (w3843:string)
                        n2552 = call "Event Log.vi"("Content"=w3840, "EVENT LOG"=w3843) -> ("EVENT LOG"=w3842:string)  [unwired: 8 in, 1 out]
                        n2553 = local write "EVENT LOG"(w3842) -> ()
                      }
                      frame #8 {
                        n2554 = Wait (ms)(milliseconds to wait=u32 50) -> ()  [unwired: 1 out]
                      }
                      frame #9 {
                        n2555 = local read "tested by"() -> (w3845:string)
                        n2556 = Concatenate Strings("Tested By :" ("Content"), w3845) -> (w3846:string)
                        n2557 = local read "EVENT LOG"() -> (w3849:string)
                        n2558 = call "Event Log.vi"("Content"=w3846, "EVENT LOG"=w3849) -> ("EVENT LOG"=w3848:string)  [unwired: 8 in, 1 out]
                        n2559 = local write "EVENT LOG"(w3848) -> ()
                      }
                      frame #10 {
                        n2560 = Wait (ms)(milliseconds to wait=u32 50) -> ()  [unwired: 1 out]
                      }
                      frame #11 {
                        n2561 = local read "TEST STANDARD"() -> (w3852:T3)
                        n2562 = case shown="\"ASTM D6079\", Default" w3852 {
                          tunnel: ["ASTM D6079" "ISO 12156" "CEC F-096-A-06" "Custom"] -> w3851
                          frame "ASTM D6079", Default {
                          }
                          frame "ISO 12156" {
                          }
                          frame "CEC F-096-A-06" {
                          }
                          frame "Custom" {
                          }
                        }
                        n2563 = Concatenate Strings("Test Standard :" ("Content"), w3851) -> (w3853:string)
                        n2564 = local read "EVENT LOG"() -> (w3856:string)
                        n2565 = call "Event Log.vi"("Content"=w3853, "EVENT LOG"=w3856) -> ("EVENT LOG"=w3855:string)  [unwired: 8 in, 1 out]
                        n2566 = local write "EVENT LOG"(w3855) -> ()
                      }
                      frame #12 {
                        n2567 = Wait (ms)(milliseconds to wait=u32 50) -> ()  [unwired: 1 out]
                      }
                      frame #13 {
                        n2568 = local read "Fuel Discription :"() -> (w3862:string)
                        n2569 = Concatenate Strings("Fuel Description :" ("Content"), w3862) -> (w3863:string)
                        n2570 = local read "EVENT LOG"() -> (w3866:string)
                        n2571 = call "Event Log.vi"("Content"=w3863, "EVENT LOG"=w3866) -> ("EVENT LOG"=w3865:string)  [unwired: 8 in, 1 out]
                        n2572 = local write "EVENT LOG"(w3865) -> ()
                      }
                      frame #14 {
                        n2573 = Wait (ms)(milliseconds to wait=u32 50) -> ()  [unwired: 1 out]
                      }
                      frame #15 {
                        n2574 = local read "Remarks :"() -> (w3868:string)
                        n2575 = Concatenate Strings("Remarks :" ("Content"), w3868) -> (w3869:string)
                        n2576 = local read "EVENT LOG"() -> (w3872:string)
                        n2577 = call "Event Log.vi"("Content"=w3869, "EVENT LOG"=w3872) -> ("EVENT LOG"=w3871:string)  [unwired: 8 in, 1 out]
                        n2578 = local write "EVENT LOG"(w3871) -> ()
                      }
                      frame #16 {
                        n2579 = Wait (ms)(milliseconds to wait=u32 50) -> ()  [unwired: 1 out]
                      }
                      frame #17 {
                        n2580 = local read "Operator ID"() -> (w3874:string)
                        n2581 = Concatenate Strings("Operator ID :" ("Content"), w3874) -> (w3876:string)
                        n2582 = local read "EVENT LOG"() -> (w3878:string)
                        n2583 = call "Event Log.vi"("Content"=w3876, "EVENT LOG"=w3878) -> ("EVENT LOG"=w3877:string)  [unwired: 8 in, 1 out]
                        n2584 = local write "EVENT LOG"(w3877) -> ()
                      }
                      frame #18 {
                        n2585 = Wait (ms)(milliseconds to wait=u32 50) -> ()  [unwired: 1 out]
                      }
                      frame #19 {
                        n2586 = disable-structure shown="Disabled" {
                          frame Disabled {
                            n2587 = local read "EVENT LOG"() -> (w3882:string)
                            n2588 = call "Event Log.vi"("Content"="Test Parameter", "EVENT LOG"=w3882) -> ("EVENT LOG"=w3881:string)  [unwired: 8 in, 1 out]
                            n2589 = local write "EVENT LOG"(w3881) -> ()
                          }
                          frame Enabled {
                          }
                        }
                      }
                      frame #20 {
                        n2590 = Wait (ms)(milliseconds to wait=u32 50) -> ()  [unwired: 1 out]
                      }
                      frame #21 {
                        n2591 = local read "Set Hz"() -> (w3886:dbl)
                        n2592 = Number To Fractional String(number=w3886, precision (6)=i16 2) -> (F-format string=w3885:string)  [unwired: 2 in]
                        n2593 = Concatenate Strings("Set Frequency [Hz] :" ("Content"), w3885) -> (w3888:string)
                        n2594 = local read "EVENT LOG"() -> (w3890:string)
                        n2595 = call "Event Log.vi"("Content"=w3888, "EVENT LOG"=w3890) -> ("EVENT LOG"=w3889:string)  [unwired: 8 in, 1 out]
                        n2596 = local write "EVENT LOG"(w3889) -> ()
                      }
                      frame #22 {
                        n2597 = Wait (ms)(milliseconds to wait=u32 50) -> ()  [unwired: 1 out]
                      }
                      frame #23 {
                        n2598 = local read "NORMAL LOAD"() -> (w3893:dbl)
                        n2599 = Number To Fractional String(number=w3893, precision (6)=i16 2) -> (F-format string=w3894:string)  [unwired: 2 in]
                        n2600 = Concatenate Strings("Applied Load [grams] :" ("Content"), w3894) -> (w3896:string)
                        n2601 = local read "EVENT LOG"() -> (w3898:string)
                        n2602 = call "Event Log.vi"("Content"=w3896, "EVENT LOG"=w3898) -> ("EVENT LOG"=w3897:string)  [unwired: 8 in, 1 out]
                        n2603 = local write "EVENT LOG"(w3897) -> ()
                      }
                      frame #24 {
                        n2604 = Wait (ms)(milliseconds to wait=u32 50) -> ()  [unwired: 1 out]
                      }
                      frame #25 {
                        n2605 = local read "Set Strk"() -> (w3901:dbl)
                        n2606 = Number To Fractional String(number=w3901, precision (6)=i16 2) -> (F-format string=w3902:string)  [unwired: 2 in]
                        n2607 = Concatenate Strings("Set Stroke [mm] :" ("Content"), w3902) -> (w3904:string)
                        n2608 = local read "EVENT LOG"() -> (w3906:string)
                        n2609 = call "Event Log.vi"("Content"=w3904, "EVENT LOG"=w3906) -> ("EVENT LOG"=w3905:string)  [unwired: 8 in, 1 out]
                        n2610 = local write "EVENT LOG"(w3905) -> ()
                      }
                      frame #26 {
                        n2611 = Wait (ms)(milliseconds to wait=u32 50) -> ()  [unwired: 1 out]
                      }
                      frame #27 {
                        n2612 = local read "Set Temp"() -> (w3909:dbl)
                        n2613 = Number To Fractional String(number=w3909, precision (6)=i16 2) -> (F-format string=w3910:string)  [unwired: 2 in]
                        n2614 = Concatenate Strings("Set Temperature [deg C] :" ("Content"), w3910) -> (w3912:string)
                        n2615 = local read "EVENT LOG"() -> (w3914:string)
                        n2616 = call "Event Log.vi"("Content"=w3912, "EVENT LOG"=w3914) -> ("EVENT LOG"=w3913:string)  [unwired: 8 in, 1 out]
                        n2617 = local write "EVENT LOG"(w3913) -> ()
                      }
                      frame #28 {
                        n2618 = Wait (ms)(milliseconds to wait=u32 50) -> ()  [unwired: 1 out]
                      }
                      frame #29 {
                        n2619 = local read "Set Rh"() -> (w3917:dbl)
                        n2620 = Number To Fractional String(number=w3917, precision (6)=i16 2) -> (F-format string=w3918:string)  [unwired: 2 in]
                        n2621 = Concatenate Strings("Set Humidity [%RH] :" ("Content"), w3918) -> (w3920:string)
                        n2622 = local read "EVENT LOG"() -> (w3922:string)
                        n2623 = call "Event Log.vi"("Content"=w3920, "EVENT LOG"=w3922) -> ("EVENT LOG"=w3921:string)  [unwired: 8 in, 1 out]
                        n2624 = local write "EVENT LOG"(w3921) -> ()
                      }
                      frame #30 {
                        n2625 = Wait (ms)(milliseconds to wait=u32 50) -> ()  [unwired: 1 out]
                      }
                      frame #31 {
                        n2626 = local read "test time"() -> (w3925:dbl)
                        n2627 = Number To Fractional String(number=w3925, precision (6)=i16 1) -> (F-format string=w3926:string)  [unwired: 2 in]
                        n2628 = Concatenate Strings("Test Duration [mins] :" ("Content"), w3926) -> (w3928:string)
                        n2629 = local read "EVENT LOG"() -> (w3930:string)
                        n2630 = call "Event Log.vi"("Content"=w3928, "EVENT LOG"=w3930) -> ("EVENT LOG"=w3929:string)  [unwired: 8 in, 1 out]
                        n2631 = local write "EVENT LOG"(w3929) -> ()
                      }
                      frame #32 {
                        w3931 = dbl[] [] ("History Data")
                        w3932 = cluster{"y":dbl, dbl, "y":dbl}[] [] ("History Data")
                        w3933 = FALSE ("Visible")
                        n2632 = property on="Stroke ( mm )" class="WFChart (strict)"("History Data"=w3932) -> ()  [unwired: 2 in, 2 out]
                        n2633 = property on="Humidity ( %RH )" class="WFChart (strict)"("History Data"=w3931) -> ()  [unwired: 2 in, 2 out]
                        n2634 = property on="Temperature ( Deg C )" class="WFChart (strict)"("History Data"=w3931) -> ()  [unwired: 2 in, 2 out]
                        n2635 = property on="Electrical Contact Resistance ( % )" class="WFChart (strict)"("History Data"=w3931) -> ()  [unwired: 2 in, 2 out]
                        n2636 = property on="Coefficient of Friction" class="WFChart (strict)"("History Data"=w3931) -> ()  [unwired: 2 in, 2 out]
                        n2637 = property on="Frictional Force ( N )" class="WFChart (strict)"("History Data"=w3931) -> ()  [unwired: 2 in, 2 out]
                        n2638 = property on="Coefficient of Friction" class="WFChart (strict)"("History Data"=w3931) -> ()  [unwired: 2 in, 2 out]
                        n2639 = property on="Frictional Force ( N )" class="WFChart (strict)"("History Data"=w3931) -> ()  [unwired: 2 in, 2 out]
                        n2640 = property on="Electrical Contact Resistance ( % )" class="WFChart (strict)"("History Data"=w3931) -> ()  [unwired: 2 in, 2 out]
